vi "ArduinoSensorFileWriteTest.vi"() -> ()   [LabVIEW 2022 SP3]
uses:
  <vilib>/Instr/_visa.llb/VISA Configure Serial Port (Instr).vi
  <vilib>/Utility/file.llb/Write Delimited Spreadsheet (string).vi
  <vilib>/Utility/file.llb/Write Delimited Spreadsheet (DBL).vi
panel:
  in  "String":string="python main.py"
  in  "Path":path=path "z:/Documents/Academics/EE491/Game"
  in  "Launch Python":bool
  in  "Channel Names":string[](array[string])=["t_val", "chan1", "chan2", "chan3", "chan4", "chan5"]
  in  "file path (dialog if empty)":path=path "\\\\Mac\\Home/Documents/Academics/EE491/data2.csv"
  in  "stop":bool
  out "Waveform Chart":dbl[][](graph)
  in  "baud rate (115200)":u32=115200
  in  "VISA resource name":refnum<visa-resource-name>
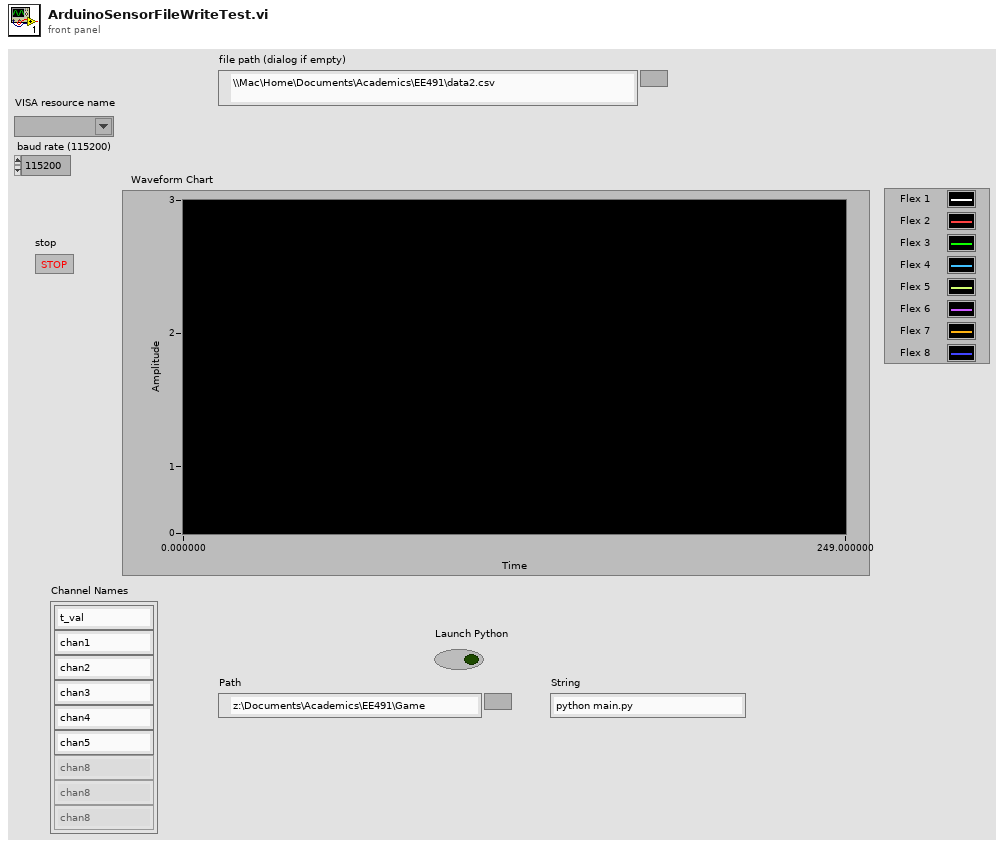
[diagram p1: front panel]
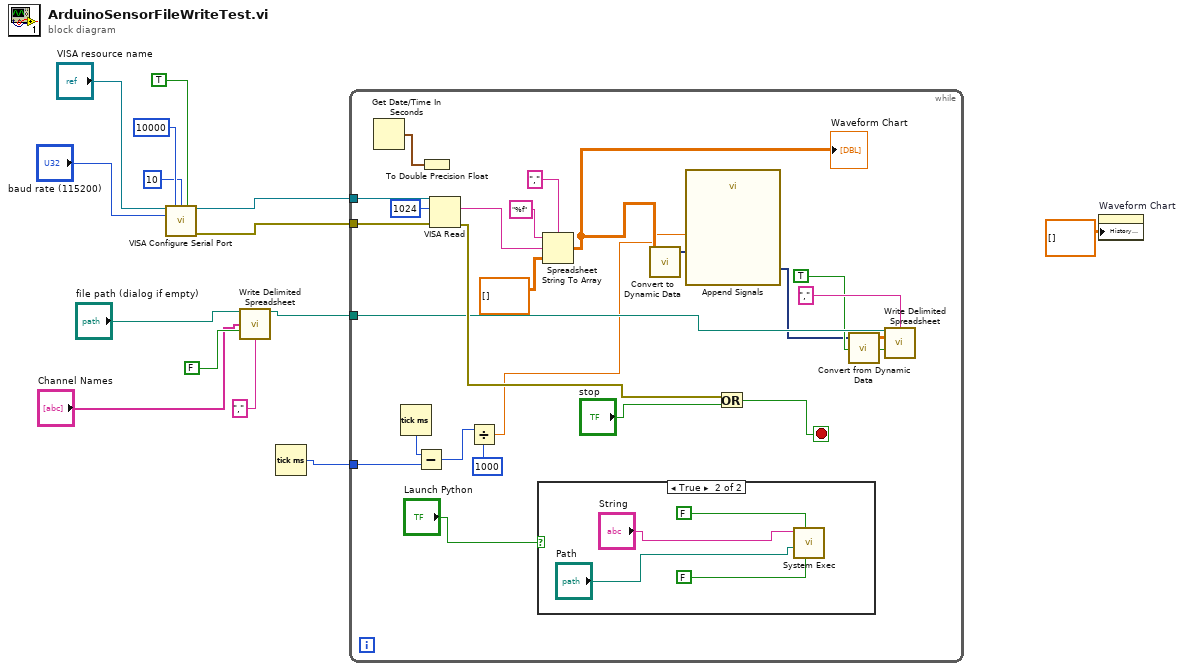
[diagram p0: block diagram]
diagram:
  n1 = call-poly "VISA Configure Serial Port"("VISA resource name"="VISA resource name", "timeout (10sec)"=u32 10000, "termination char\n(0xA = '\\n' = LF)"=u8 10 ("termination char\n(0xA = '\\n' = LF)"), "Enable Termination\nChar (T)"=TRUE ("Enable Termination\nChar (T)"), "baud rate (9600)"="baud rate (115200)") -> ("VISA resource name out"=w14:refnum<visa-resource-name>, "error out"=w13:errorcluster)  [unwired: 9 in]
  n2 = call-poly <vilib>:"Write Delimited Spreadsheet.vi"("file path (dialog if empty)"="file path (dialog if empty)", "1D data"="Channel Names", "append to file? (new file:F)"=FALSE, "delimiter (\\t)"="," ("delimiter (\\t)")) -> ("new file path (Not A Path if cancelled)"=w7:path)  [unwired: 10 in, 1 out]
  n3 = Tick Count (ms)() -> (millisecond timer value=w2:u32)
  n4 = while {
    tunnel: w14 -> [w38]
    tunnel: w13 -> [w37]
    tunnel: w7 -> [w28]
    tunnel: w2 -> [w18]
    stop <- w31 stop-if-true
    n5 = Get Date/Time In Seconds() -> (seconds since 1Jan1904=w21:timestamp)
    n6 = Tick Count (ms)() -> (millisecond timer value=w19:u32)
    n7 = Subtract(x=w19, y=w18) -> (x-y=w17:u32)
    n8 = To Double Precision Float(number=w21) -> ()  [unwired: 1 out]
    n9 = VISA Read(VISA resource name=w38, byte count=u32 1024, error in (no error)=w37) -> (read buffer=w35:string, error out=w29:errorcluster)  [unwired: 2 out]
    n10 = Divide(x=w17, y=u32 1000) -> (x/y=w15:dbl)
    n11 = case shown="True" "Launch Python" {
      frame False {
      }
      frame True {
        n12 = call <vilib>:"System Exec.vi"("run minimized? (F)"=FALSE, "wait until completion? (T)"=FALSE, "working directory"="Path", "command line"="String") -> ()  [unwired: 4 in, 4 out]
      }
    }
    n13 = Spreadsheet String To Array(delimiter (Tab)=",", format string="%f", spreadsheet string=w35, array type (2D Dbl)=dbl[][] []) -> (array=w25:dbl[][])
    "Waveform Chart" <- w25
    n14 = call "Convert to Dynamic Data"("2D Array"=w25) -> ("Dynamic Data Type"=w24:dynamicdata)  [unwired: 3 in]
    n15 = call "Append Signals"("Input Signal B"=w24, "Input Signal A"=w15) -> ("Appended Signals"=w23:dynamicdata)  [unwired: 8 in, 1 out]
    n16 = Or(x=w29, y="stop") -> (x .or. y?=w31:bool)
    n17 = call "Convert from Dynamic Data"("Dynamic Data Type"=w23) -> ("Array"=w22:dbl[][])  [unwired: 3 in]
    n18 = call-poly <vilib>:"Write Delimited Spreadsheet.vi"("file path (dialog if empty)"=w28, "2D data"=w22, "append to file? (new file:F)"=TRUE, "delimiter (\\t)"="," ("delimiter (\\t)")) -> ()  [unwired: 10 in, 2 out]
  }
  n19 = property on="Waveform Chart" class="WFChart (strict)"("History Data"=dbl[][] []) -> ()  [unwired: 2 in, 2 out]
